vi "TitlePrompt.vi"(0 "Title":string) -> (1 "Cancelled":bool, 2 "Title Out":string)   [LabVIEW 2014]
panel:
  in  "Cancel":bool
  in  "OK":bool
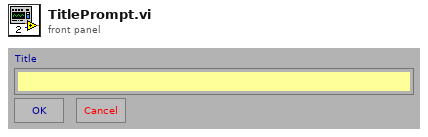
[diagram p1: front panel]
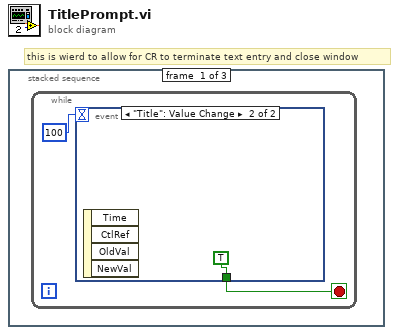
[diagram p0: block diagram]
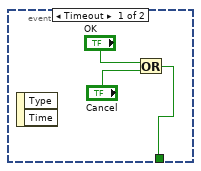
[diagram p2: hidden frame]
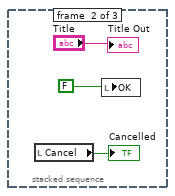
[diagram p3: hidden frame]
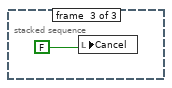
[diagram p4: hidden frame]
diagram:
  # "this is wierd to allow for CR to terminate text entry and close window"
  n1 = stacked-sequence {
    frame #0 {
      n2 = while {
        stop <- w1 stop-if-true
        n3 = event shown="[1] \"Title\": Value Change" {
          selector: _ -> [_ _]
          dyn-events: _ -> [_ _]
          timeout: 100 -> [_ _]
          tunnel: [w3 TRUE ("OK")] -> w1
          event Timeout {
            n4 = event-data() -> ()  [unwired: 1 in, 2 out]
            n5 = Or(x="OK", y="Cancel") -> (x .or. y?=w3:bool)
          }
          event "Title": Value Change {
            n6 = event-data() -> ()  [unwired: 1 in, 4 out]
          }
        }
      }
    }
    frame #1 {
      n7 = local read "Cancel"() -> (→"Cancelled":bool)
      n8 = local write "OK"(FALSE ("OK")) -> ()
      "Title Out" <- "Title"
    }
    frame #2 {
      n9 = local write "Cancel"(FALSE ("Cancel")) -> ()
    }
  }
